vi "Get Actor.vi"(11 "Dev Actor in":refnum<class "Dev Actor.lvclass">) -> (2 "Actor":refnum<class "Actor.lvclass">)   [LabVIEW 2021, in "Dev Actor.lvlib" / "Dev Actor.lvclass"]
uses:
  <vilib>/jettl/jettl/Actor/Actor/Actor.lvclass
  Dev Actor.lvclass
  Dev Actor.lvclass/Dev Actor.ctl
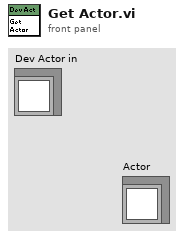
[diagram p1: front panel]
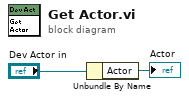
[diagram p0: block diagram]
diagram:
  n1 = Unbundle By Name("Dev Actor in") -> ("Actor"=→"Actor":refnum<class "Actor.lvclass">)
